vi "copy file in.vi"(8 "error in (no error)":errorcluster, 10 "selected path":path, 11 "device_type in":refnum<class "device_type.lvclass">) -> (0 "error out":errorcluster, 2 "number of pulses":dbl, 3 "device_type out":refnum<class "device_type.lvclass">)   [LabVIEW 2021, in "device_type.lvclass"]
uses:
  device_type.lvclass
  device_type.lvclass/device_type.ctl
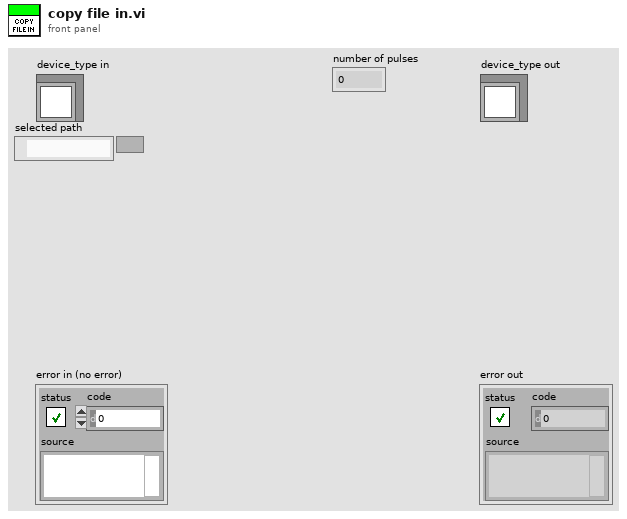
[diagram p1: front panel]
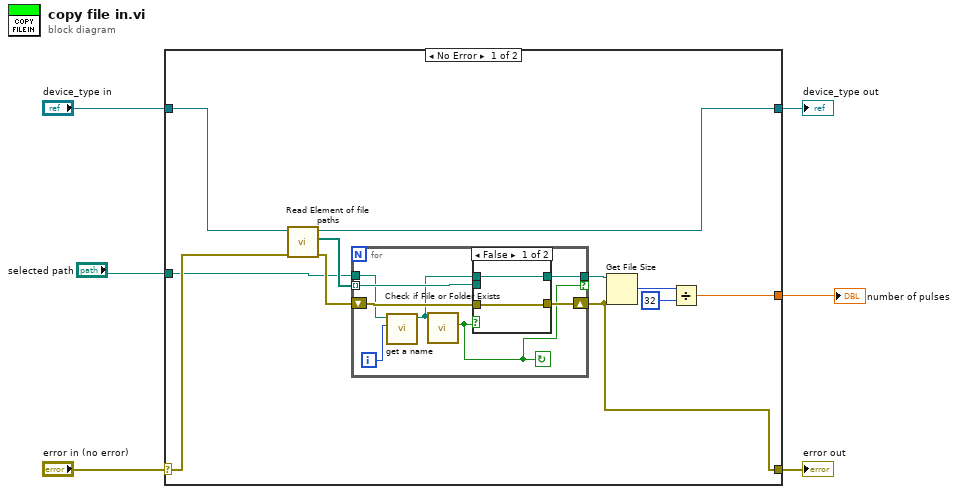
[diagram p0: block diagram]
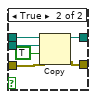
[diagram p2: hidden frame]
diagram:
  n1 = case shown="No Error" "error in (no error)" {
    selector: "error in (no error)" -> [w11 w35]
    tunnel: [w8 w35] -> w5
    tunnel: [w9 w34] -> w3
    tunnel: "device_type in" -> [w12 w34]
    tunnel: "selected path" -> [w10 _]
    tunnel: [w7 _] -> w1
    frame No Error {
      n2 = call-dynamic "Read Element of file paths.vi"("error in (no error)"=w11, "device_type in"=w12) -> ("error out"=w16:errorcluster, "file paths"=w17:path[], "device_type out"=w9:refnum<class "device_type.lvclass">)  [unwired: 7 in]
      n3 = for {
        tunnel: w10 -> [w20]
        tunnel: w17 -> [w25] mode=indexing
        shift-right: [w23] -> w8
        shift-left: w16 -> [w24]
        tunnel: [w22] -> w15 if=w18
        i -> [w21]
        stop <- w18 continue-if-true
        n4 = call "get a name.vi"("Numeric"=w21, "Bitfile path"=w20) -> ("Path"=w19:path)  [unwired: 8 in, 1 out]
        n5 = call <vilib>:"Check if File or Folder Exists.vi"("path"=w19) -> ("file or folder exists?"=w18:bool)  [unwired: 8 in, 2 out]
        n6 = case shown="False" w18 {
          tunnel: w25 -> [_ w33]
          tunnel: w24 -> [w27 w31]
          tunnel: [w27 w30] -> w23
          tunnel: [w26 w29] -> w22
          tunnel: w19 -> [w26 w28]
          frame False {
          }
          frame True {
            n7 = Copy(8:w31, 9:TRUE ("overwrite (F)"), 10:w33, 11:w28) -> (0:w30:errorcluster, 3:w29:path)  [unwired: 1 in, 1 out]
          }
        }
      }
      n8 = Get File Size(file=w15, error in=w8) -> (size (in bytes)=w14:i64)  [unwired: 2 out]
      n9 = Divide(x=w14, y=i64 32) -> (x/y=w7:dbl)
    }
    frame Error {
    }
  }
  "error out" <- w5
  "device_type out" <- w3
  "number of pulses" <- w1
